vi "SampleClient.vi"() -> ()   [LabVIEW 2012]
panel:
  out "Simulation UDP":bool
  out "Position UDP":bool
  out "Robot Y":i32
  out "Robot X":i32
  out "Setup Running?":bool
  out "error out":errorcluster
  out "Heading":i32
  in  "Right PWM Value":i32=1500
  in  "Left PWM Value":i32=1500
  in  "stop":bool
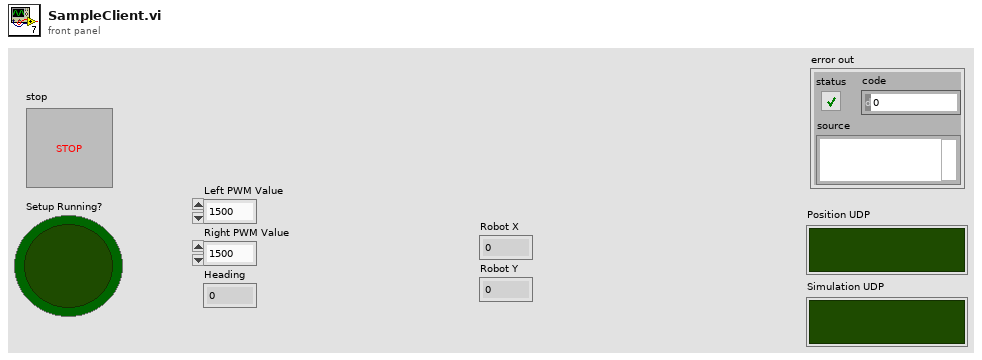
[diagram p1: front panel]
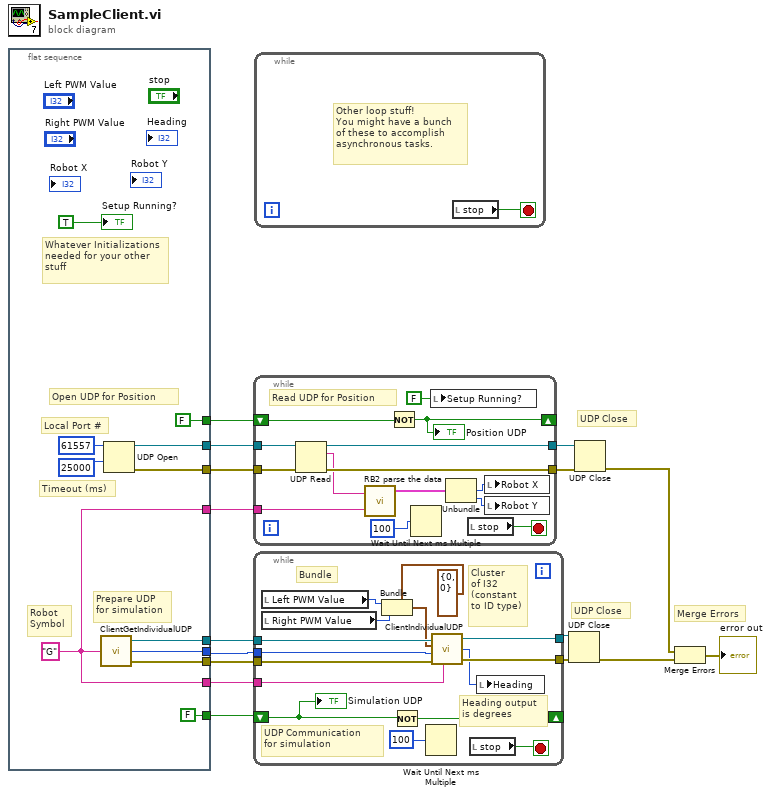
[diagram p0: block diagram]
diagram:
  # "Merge Errors"
  # "UDP Close"
  # "UDP Close"
  n1 = flat-sequence {
    tunnel: [w27] -> w14
    tunnel: [w26] -> w13
    tunnel: [w25] -> w15
    tunnel: [w23] -> w16
    tunnel: [w23] -> w10
    tunnel: [w21] -> w9
    tunnel: [w20] -> w8
    tunnel: [FALSE] -> w2
    tunnel: [FALSE] -> w1
    frame #0 {
      w23 = "G"
      # "Prepare UDP\nfor simulation"
      # "Timeout (ms)"
      # "Local Port #"
      # "Open UDP for Position"
      # "Whatever Initializations\nneeded for your other\nstuff"
      # "Robot \nSymbol"
      n2 = call "ClientGetIndividualUDP.vi"("Robot Symbol"=w23) -> ("UDP Connection ID"=w27:refnum<k16>, "Remote Port #"=w26:i32, "error out"=w25:errorcluster)
      n3 = UDP Open(9:25000 ("timeout ms (25000)"), 11:u16 61557 ("port")) -> (port=w20:refnum<k16>, 0:w21:errorcluster)  [unwired: 3 in, 1 out]
      "Setup Running?" <- TRUE
    }
  }
  n4 = while {
    tunnel: w10 -> [w41]
    tunnel: w9 -> [w35]
    tunnel: w8 -> [w36]
    tunnel: [w34] -> w7
    tunnel: [w33] -> w6
    shift-right: [w29] -> _
    shift-left: w1 -> [w30]
    stop <- w37 stop-if-true
    # "Read UDP for Position"
    n5 = UDP Read(connection ID=w36, 8:w35) -> (data out=w32:string, error out=w33:errorcluster, 3:w34:refnum<k16>)  [unwired: 2 in, 2 out]
    n6 = call "RB2 parse the data.vi"("Nav String"=w32, "Jeep"=w41) -> ("Jeep Data"=w40:cluster{"Header":string, i32, i32})  [unwired: 2 out]
    n7 = Not(x=w30) -> (.not. x?=w29:bool)
    "Position UDP" <- w29
    n8 = Wait Until Next ms Multiple(millisecond multiple=u32 100) -> ()  [unwired: 1 out]
    n9 = local write "Setup Running?"(FALSE ("Setup Running?")) -> ()
    n10 = Unbundle(w40) -> (w39:i32, w38:i32)  [unwired: 1 out]
    n11 = local read "stop"() -> (w37:bool)
    n12 = local write "Robot X"(w39) -> ()
    n13 = local write "Robot Y"(w38) -> ()
  }
  n14 = while {
    tunnel: w16 -> [w56]
    tunnel: w15 -> [w55]
    tunnel: w14 -> [w54]
    tunnel: w13 -> [w53]
    tunnel: [w48] -> w11
    tunnel: [w47] -> w12
    shift-right: [w44] -> _
    shift-left: w2 -> [w43]
    stop <- w45 stop-if-true
    # "UDP Communication \nfor simulation"
    # "Heading output\nis degrees"
    # "Cluster\nof I32\n(constant\nto ID type)"
    # "Bundle"
    n15 = local read "Left PWM Value"() -> (w52:i32)
    n16 = local read "Right PWM Value"() -> (w51:i32)
    n17 = Bundle(cluster=cluster{i32, i32} {0, 0}, w52, w51) -> (w50:cluster{i32, i32})
    n18 = Not(x=w43) -> (.not. x?=w44:bool)
    n19 = Wait Until Next ms Multiple(millisecond multiple=u32 100) -> ()  [unwired: 1 out]
    n20 = call "ClientIndividualUDP.vi"("UDP Connection ID"=w54, "Rover Inputs"=w50, "Remote Port #"=w53, "error in (no error)"=w55, "Robot Symbol"=w56) -> ("connection ID out"=w48:refnum<k16>, "Robot Heading"=w46:i32, "error out"=w47:errorcluster)
    n21 = local read "stop"() -> (w45:bool)
    n22 = local write "Heading"(w46) -> ()
    "Simulation UDP" <- w43
  }
  n23 = while {
    stop <- w57 stop-if-true
    # "Other loop stuff!\nYou might have a bunch\nof these to accomplish\nasynchronous tasks."
    n24 = local read "stop"() -> (w57:bool)
  }
  n25 = UDP Close(connection ID=w11, 8:w12) -> (error out=w4:errorcluster)  [unwired: 1 out]
  n26 = UDP Close(connection ID=w7, 8:w6) -> (error out=w3:errorcluster)  [unwired: 1 out]
  n27 = Merge Errors(w3, w4) -> (→"error out":errorcluster)
